vi "switch file to cluster.vi"() -> ()   [LabVIEW 2015, in "SLSC Switch.lvclass"]
uses:
  SLSC Switch.lvclass
panel:
  in  "shw path":path
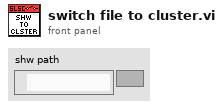
[diagram p1: front panel]
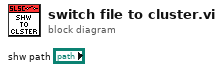
[diagram p0: block diagram]
diagram:
